vi "Text File Reader Test.vi"() -> ()   [LabVIEW 2014]
panel:
  out "Array of Strings":string[](array[string])
  out "text":string
  out "lowercase file extension":string
  out "creator":string
  out "type":string
  out "selected path":path
  in  "Open Button":bool
  in  "Stop Button":bool
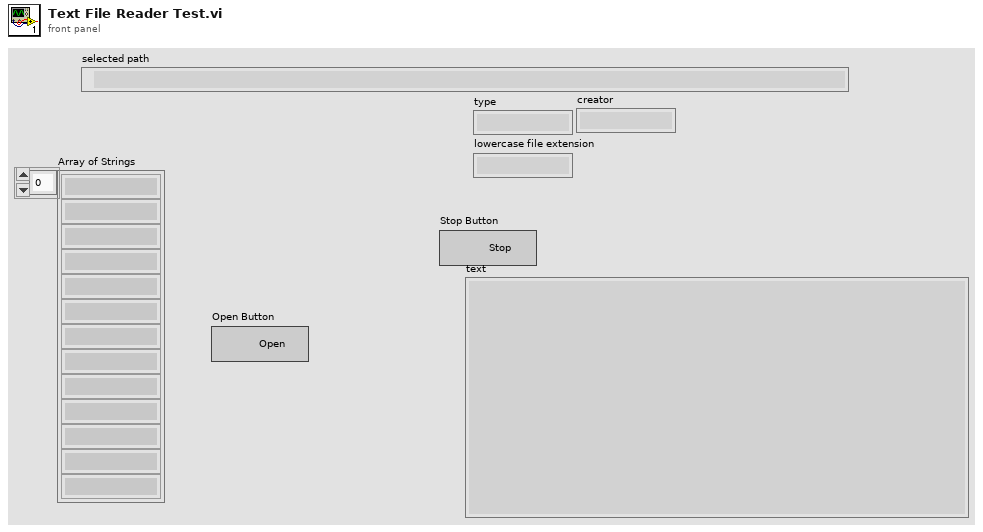
[diagram p1: front panel]
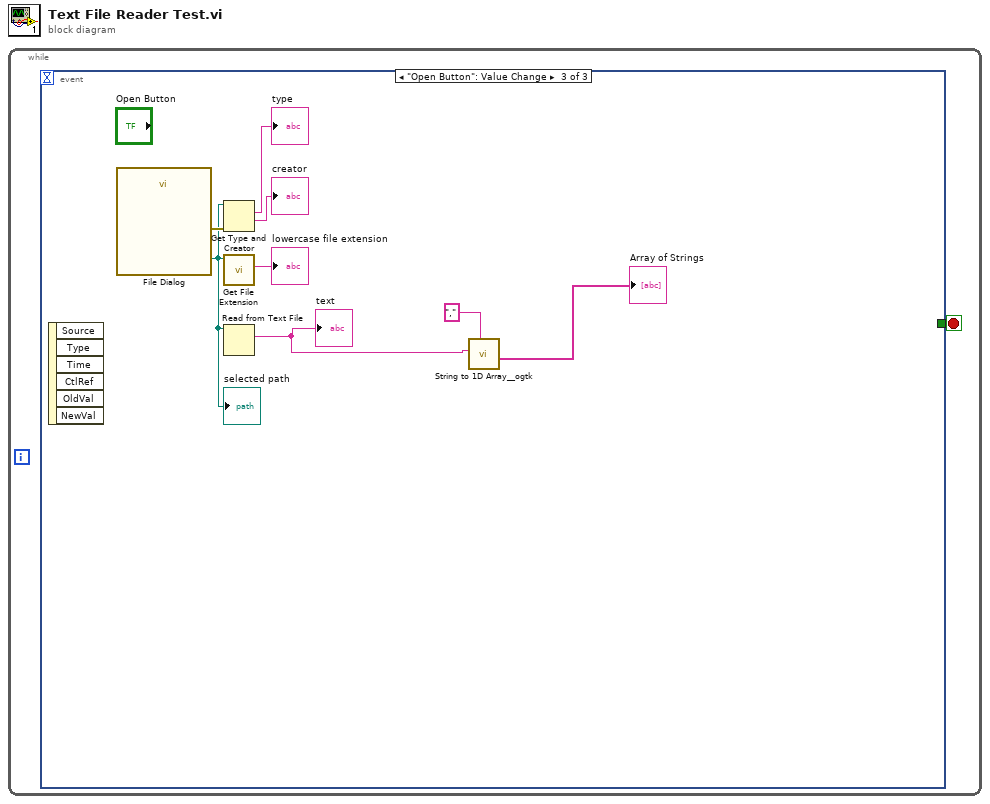
[diagram p0: block diagram]
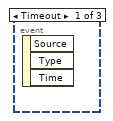
[diagram p2: hidden frame]
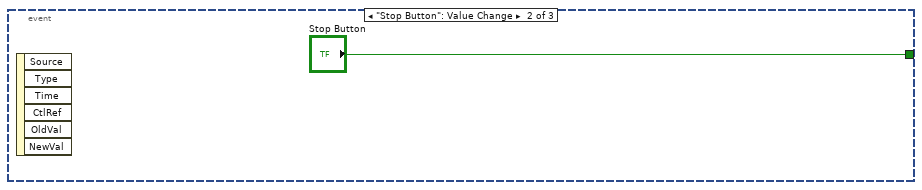
[diagram p3: hidden frame]
diagram:
  n1 = while {
    stop <- w1 stop-if-true
    n2 = event shown="[2] \"Open Button\": Value Change" {
      selector: _ -> [_ _ _]
      dyn-events: _ -> [_ _ _]
      timeout: _ -> [_ _ _]
      tunnel: [_ "Stop Button" _] -> w1
      event Timeout {
        n3 = event-data() -> ()  [unwired: 1 in, 3 out]
      }
      event "Stop Button": Value Change {
        n4 = event-data() -> ()  [unwired: 1 in, 6 out]
      }
      event "Open Button": Value Change {
        n5 = event-data() -> ()  [unwired: 1 in, 6 out]
        n6 = call "File Dialog"() -> ("selected path"=w6:path, "error out"=w10:errorcluster)  [unwired: 12 in, 2 out]
        "selected path" <- w6
        n7 = Get Type and Creator(4:w10, 7:w6) -> (1:→"creator":string, 2:→"type":string)  [unwired: 2 out]
        n8 = call <vilib>:"Get File Extension.vi"("file"=w6) -> ("lowercase file extension"=→"lowercase file extension":string)  [unwired: 7 in, 3 out]
        n9 = Read from Text File(file (use dialog)=w6) -> (text=w5:string)  [unwired: 3 in, 3 out]
        "text" <- w5
        n10 = call <userlib>:"String to 1D Array__ogtk.vi"("delimiter (Tab)"=",", "string"=w5) -> ("Array of Strings"=→"Array of Strings":string[])  [unwired: 9 in]
      }
    }
  }
